vi "Get Buffer Status.vi"(8 "error in":errorcluster, 11 "Buffer in":refnum<data-value>) -> (0 "error out":errorcluster, 1 "bufSize":i32, 2 "nbElements":i32, 3 "Buffer":refnum<data-value>, 4 "full":bool)   [LabVIEW 2013, in "CircularBuffer.lvlib" / "VariantBuffer.lvclass"]
doc: "This VI returns data from the ring buffer starting from the oldest data and ending with the newest.\n\nThe data is duplicated at the output so this VI allocates new place in the memory for the output."
uses:
  VariantBuffer.lvclass
  VariantBuffer.lvclass/VariantBuffer.ctl
  WriteBufferError.vi
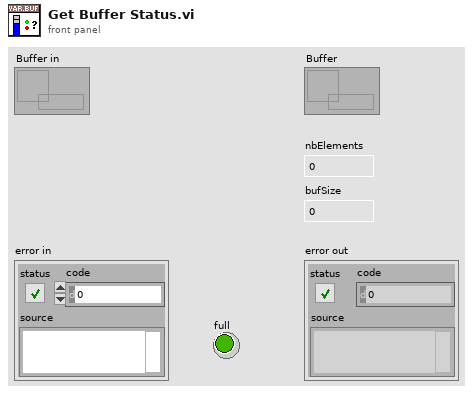
[diagram p1: front panel]
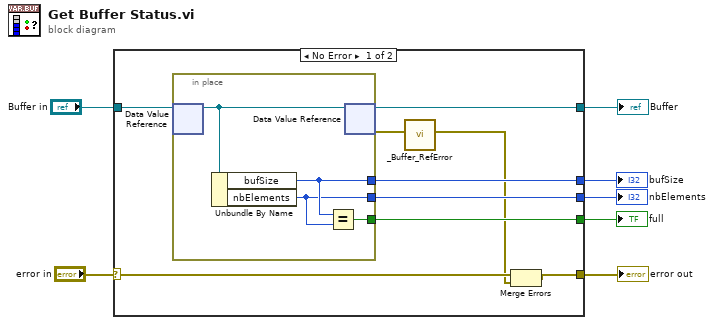
[diagram p0: block diagram]
diagram:
  n1 = case shown="No Error" "error in" {
    selector: "error in" -> [w12 w21]
    tunnel: "Buffer in" -> [w16 w22]
    tunnel: [w15 w22] -> w6
    tunnel: [w14 w21] -> w3
    tunnel: [w13 _] -> w5
    tunnel: [w11 _] -> w2
    tunnel: [w10 _] -> w1
    frame No Error {
      n2 = in-place {
        in-place-border: [w19] -> w13
        in-place-border: [w20] -> w11
        in-place-border: [w18] -> w10
        n3 = in-place-dvr #1(w16) -> (w17:refnum<class "VariantBuffer.lvclass">)  [unwired: 1 out]
        n4 = Unbundle By Name(w17) -> ("bufSize"=w20:i32, "nbElements"=w19:i32)
        n5 = Equal?(x=w20, y=w19) -> (x = y?=w18:bool)
        n6 = in-place-dvr #1(w17) -> (w15:refnum<data-value>, w9:errorcluster)
      }
      n7 = call "_Buffer_RefError.vi"("error in (no error)"=w9) -> ("error out"=w8:errorcluster)  [unwired: 10 in]
      n8 = Merge Errors(w12, w8) -> (w14:errorcluster)
    }
    frame Error {
    }
  }
  "error out" <- w3
  "Buffer" <- w6
  "nbElements" <- w5
  "bufSize" <- w2
  "full" <- w1
